vi "SetDirection.vi"(8 "error in (no error)":errorcluster, 9 "direction":i32(ring)=1 items=["Increase"=1, "Decrease"=2], 10 "channel":i32(ring)=1 items=["Channel1"=1, "Channel2"=2, "Channel3"=3, "Channel4"=4], 11 "KIM101 in":refnum<class "KIM101.lvclass">) -> (0 "error out":errorcluster, 3 "KIM101 out":refnum<class "KIM101.lvclass">)   [LabVIEW 2023, in "KIM101.lvlib" / "KIM101.lvclass"]
uses:
  KIM101.lvclass
  KIM101.lvclass/KIM101.ctl
  C:/Users/quantum/Documents/LVDAQ/UIs/TranslationStage_UI/Thorlabs.MotionControl.KCube.InertialMotorCLI.dll
  UIs/TranslationStage_UI/Thorlabs.MotionControl.KCube.InertialMotorCLI.dll
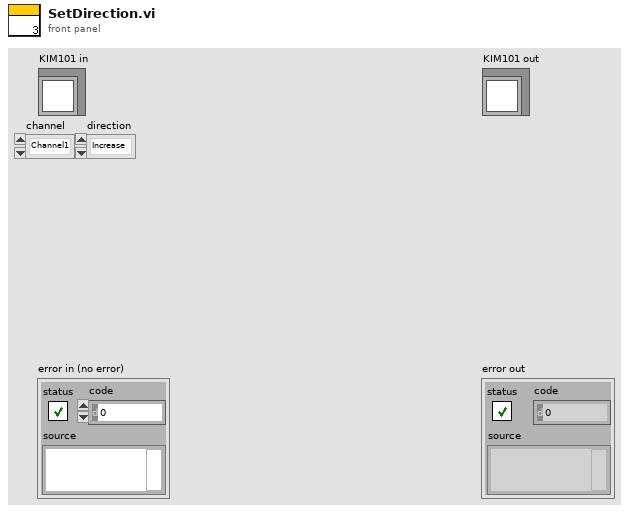
[diagram p1: front panel]
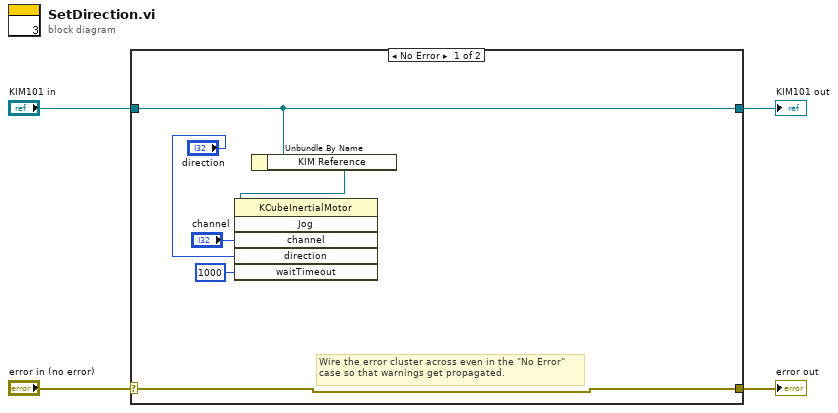
[diagram p0: block diagram]
diagram:
  n1 = case shown="No Error" "error in (no error)" {
    selector: "error in (no error)" -> [w10 w12]
    tunnel: [w10 w12] -> w3
    tunnel: [w9 w11] -> w1
    tunnel: "KIM101 in" -> [w9 w11]
    frame No Error {
      # "Wire the error cluster across even in the \"No Error\"\ncase so that warnings get propagated."
      n2 = Unbundle By Name(w9) -> ("KIM Reference"=w8:refnum<k24>)
      n3 = invoke class="KCubeInertialMotor" method="Jog"(reference=w8, "channel"="channel", "direction"="direction", "waitTimeout"=1000) -> ()  [unwired: 2 in, 6 out]
    }
    frame Error {
    }
  }
  "error out" <- w3
  "KIM101 out" <- w1
